vi "Write Value with Timestamp.vi"(7 "IgnoreIfEqual (F)":bool, 8 "error in (no error)":errorcluster, 9 "Timestamp (now)":timestamp, 10 "Value":variant, 11 "Tag in":refnum<class "Tag.lvclass">) -> (0 "error out":errorcluster, 3 "Tag out":refnum<class "Tag.lvclass">)   [LabVIEW 2018, in "Tag Engine.lvlib" / "Tag.lvclass"]
uses:
  Tag.lvclass
  Tag.lvclass/Tag.ctl
  Types/ValChange Cluster.ctl
  <vilib>/Utility/Data Type/Type Definitions/Data Type.ctl
  Tag Engine.lvlib
  <vilib>/Utility/Data Type/NI_Data Type.lvlib
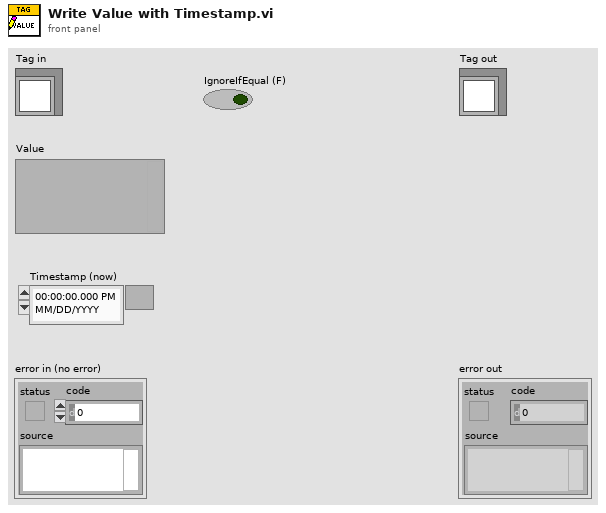
[diagram p1: front panel]
types:
  T1 = typedef "Tag Engine.lvlib/ValChange Cluster.ctl" = cluster{"Tag Name":string, "Type":T2, "Old Value":variant, "Old Time Stamp":timestamp, "New Value":variant, "New Time Stamp":timestamp}
  T2 = typedef "NI_Data Type.lvlib/Data Type.ctl" = enum8{"Invalid Type", "Void", "I8", "I16", "I32", "I64", "U8", "U16", "U32", "U64", "Single Float", "Double Float", "Extended Float", "Single Complex", "Double Complex", "Extended Complex", "Enum U8", "Enum U16", "Enum U32", "Enum U64", "Single Float With Unit", "Double Float With Unit", "Extended Float With Unit", "Single Complex with Unit", "Double Complex with Unit", "Extended Complex with Unit", "Boolean", "String", "Path", "Picture", "Tag", "Array", "Cluster", "Variant", "LV Variant", "Waveform", "Timestamp", "Digital Waveform", "Digital Data", "ExpressData", "Refnum", "External Data", "VI", "Poly VI", "LabVIEW Class Instance", "Fixed Point"}
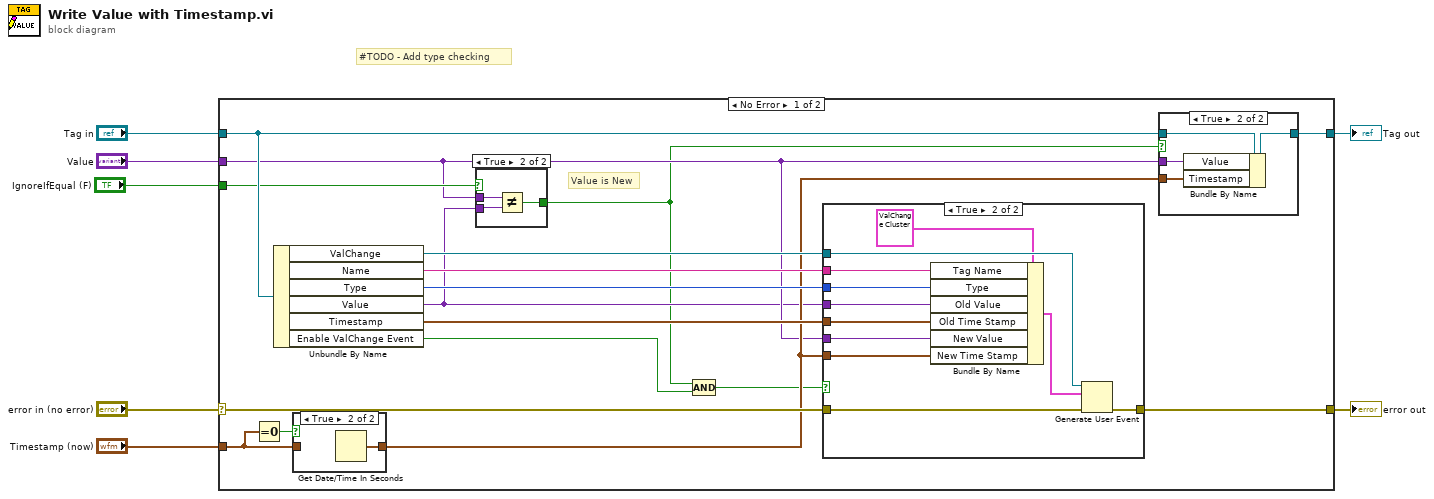
[diagram p0: block diagram]
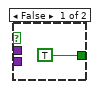
[diagram p3: hidden frame]
diagram:
  # "#TODO - Add type checking"
  n1 = case shown="No Error" "error in (no error)" {
    selector: "error in (no error)" -> [w19 w48]
    tunnel: [w18 w48] -> w6
    tunnel: [w24 w49] -> w4
    tunnel: "Tag in" -> [w23 w49]
    tunnel: "Value" -> [w12 _]
    tunnel: "Timestamp (now)" -> [w14 _]
    tunnel: "IgnoreIfEqual (F)" -> [w13 _]
    frame No Error {
      # "Value is New"
      n2 = Equal To 0?(x=w14) -> (x = 0?=w15:bool)
      n3 = Unbundle By Name(w23) -> ("ValChange"=w20:refnum<user-event>, "Name"=w22:string, "Type"=w21:T2, "Value"=w11:variant, "Timestamp"=w17:timestamp, "Enable ValChange Event"=w10:bool)
      n4 = case shown="True" w15 {
        tunnel: [w34 w35] -> w16
        tunnel: w14 -> [w34 _]
        frame False {
        }
        frame True {
          n5 = Get Date/Time In Seconds() -> (seconds since 1Jan1904=w35:timestamp)
        }
      }
      n6 = case shown="True" w13 {
        tunnel: w12 -> [_ w33]
        tunnel: w11 -> [_ w32]
        tunnel: [TRUE w31] -> w8
        frame False {
        }
        frame True {
          n7 = Not Equal?(x=w33, y=w32) -> (x != y?=w31:bool)
        }
      }
      n8 = Compound Arithmetic op=AND(w8, w10) -> (w9:bool)
      n9 = case shown="True" w9 {
        tunnel: w22 -> [_ w43]
        tunnel: w21 -> [_ w42]
        tunnel: w20 -> [_ w45]
        tunnel: w19 -> [w36 w47]
        tunnel: [w36 w46] -> w18
        tunnel: w11 -> [_ w41]
        tunnel: w17 -> [_ w40]
        tunnel: w12 -> [_ w39]
        tunnel: w16 -> [_ w38]
        frame False {
        }
        frame True {
          n10 = Bundle By Name(cluster=T1 {"Tag Name"="", "Type"=enum."Variant", "Old Value"=variant, "Old Time Stamp"=timestamp(0 s since 1904-01-01), "New Value"=variant, "New Time Stamp"=timestamp(0 s since 1904-01-01)} ("event data"), "Tag Name"=w43, "Type"=w42, "Old Value"=w41, "Old Time Stamp"=w40, "New Value"=w39, "New Time Stamp"=w38) -> (w37:T1)
          n11 = Generate User Event(user event=w45, event data cluster=w37, error in=w47) -> (error out=w46:errorcluster)  [unwired: 1 in, 1 out]
        }
      }
      n12 = case shown="True" w8 {
        tunnel: [w25 w29] -> w24
        tunnel: w23 -> [w25 w28]
        tunnel: w16 -> [_ w27]
        tunnel: w12 -> [_ w26]
        frame False {
          # "Ignore"
        }
        frame True {
          n13 = Bundle By Name(cluster=w28, "Value"=w26, "Timestamp"=w27) -> (w29:refnum<class "Tag.lvclass">)
        }
      }
    }
    frame Error {
    }
  }
  "error out" <- w6
  "Tag out" <- w4
